vi "DataPacker_Manager.vi"(7 "Request Debug Mode":bool, 8 "max queue size (-1=unlimited)":i32=10000, 9 "MIDAS Sever Port":u16=12345, 10 "MIDAS Server":string="my_midas_server.domain", 11 "Override Max Event size (Data rate bytes/s). Use MIDAS Default = 0":u32) -> ()   [LabVIEW 2018, in "feGEM DataPacker.lvlib"]
uses:
  feGEM DataPacker.lvlib
  DataPacker/DataStructures/GEM_BANK_CLUSTER_typedef.ctl
  DataPacker/DataStructures/GEM_DATA_cluster_typedef.ctl
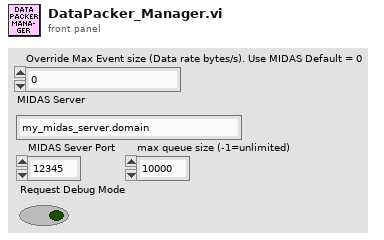
[diagram p1: front panel]
types:
  T1 = typedef "feGEM DataPacker.lvlib/GEM_BANK_CLUSTER_typedef.ctl" = cluster{"Category":string, "Variable Name":string, "Equipment description":string, "History Settings":u16, "Period to update history plots":u16, "GEM_DATA Cluster":T2}
  T2 = typedef "feGEM DataPacker.lvlib/GEM_DATA_cluster_typedef.ctl" = cluster{"DataType":string, "Formatted Data":u8[], "data byte order (Little Endian prefered)":enum16{"big-endian, network order", "native, host order", "little-endian"}}
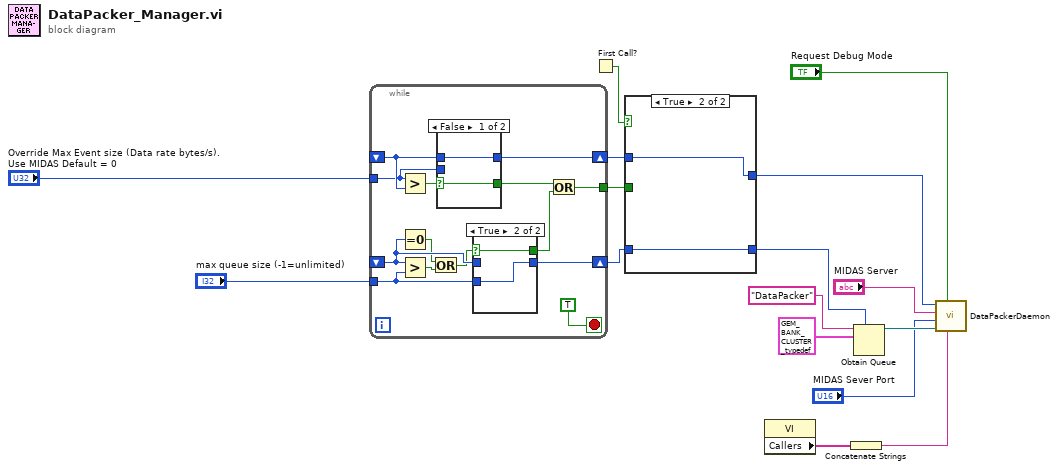
[diagram p0: block diagram]
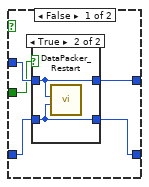
[diagram p2: hidden frame]
diagram:
  n1 = while {
    tunnel: "Override Max Event size (Data rate bytes/s). Use MIDAS Default = 0" -> [w21]
    shift-right: [w28] -> w15
    shift-left: _ -> [w22]
    tunnel: "max queue size (-1=unlimited)" -> [w27]
    shift-right: [w26] -> w13
    shift-left: _ -> [w20]
    tunnel: [w23] -> w8
    stop <- TRUE stop-if-true
    n2 = Greater?(x=w21, y=w22) -> (0:w29:bool)
    n3 = Equal To 0?(x=w20) -> (x = 0?=w19:bool)
    n4 = Greater?(x=w20, y=w27) -> (0:w18:bool)
    n5 = Or(x=w19, y=w18) -> (x .or. y?=w17:bool)
    n6 = case shown="False" w29 {
      selector: w29 -> [w35 w37]
      tunnel: w21 -> [_ w38]
      tunnel: [w36 w38] -> w28
      tunnel: w22 -> [w36 _]
      tunnel: [w35 w37] -> w25
      frame False {
      }
      frame True {
      }
    }
    n7 = case shown="True" w17 {
      selector: w17 -> [w31 w33]
      tunnel: w27 -> [_ w34]
      tunnel: [w32 w34] -> w26
      tunnel: w20 -> [w32 _]
      tunnel: [w31 w33] -> w24
      frame False {
      }
      frame True {
      }
    }
    n8 = Or(x=w25, y=w24) -> (x .or. y?=w23:bool)
  }
  n9 = First Call?() -> (First Call?: T/F=w5:bool)
  n10 = case shown="True" w5 {
    tunnel: w15 -> [w43 w49]
    tunnel: w13 -> [w42 w48]
    tunnel: w8 -> [w41 _]
    tunnel: [w40 w49] -> w7
    tunnel: [w39 w48] -> w6
    frame False {
      n11 = case shown="True" w41 {
        tunnel: w43 -> [w45 w47]
        tunnel: w42 -> [w44 w46]
        tunnel: [w45 w47] -> w40
        tunnel: [w44 w46] -> w39
        frame False {
        }
        frame True {
          n12 = call "DataPacker_Restart.vi"("Max Queue Size (-1, unlimited)"=w46, "Override Max Event size (Data rate kb/s). Use MIDAS Default = 0"=w47) -> ()  [unwired: 10 in]
        }
      }
    }
    frame True {
    }
  }
  n13 = property class="VI"() -> ("Callers"=w2:string[])  [unwired: 2 in, 2 out]
  n14 = Concatenate Strings(w2) -> (w1:string)
  n15 = Obtain Queue(max queue size (-1, unlimited)=w6, name (unnamed)="DataPacker", element data type=T1 {"Category"="", "Variable Name"="", "Equipment description"="", "History Settings"=0, "Period to update history plots"=0, "GEM_DATA Cluster"={"DataType"="", "Formatted Data"=[], "data byte order (Little Endian prefered)"=enum."big-endian, network order"}} ("output cluster")) -> (queue out=w12:refnum<queue>)  [unwired: 2 in, 2 out]
  n16 = call "DataPackerDaemon.vi"("Callers (Main VI name)"=w1, "Request Debug Mode"="Request Debug Mode", "DataPacker Queue"=w12, "MIDAS Sever Port"="MIDAS Sever Port", "MIDAS Server"="MIDAS Server", "Override Max Event size (Data rate bytes/s). Use MIDAS Default = 0"=w7) -> ()  [unwired: 5 in]
